vi "Control - Generic - Port Injection Basic Host.vi"() -> ()   [LabVIEW 2015, in "ECS-Host.lvlib"]
uses:
  ECS-Host.lvlib
  <vilib>/addons/Software Calibration Management/XControls/TBL2D.xctl
panel:
  out "InjAdv_Des":sgl[](array[numeric]) caption="[DBTDC]"
  out "InjAdv_TblOut":sgl caption="[DBTDC]"
  in  "CylFuelSplit":sgl[](array[numeric]) caption="[%]"
  in  "InjQty_ManE":bool caption="Enable Inj"
  in  "InjQty_Man":sgl caption="[mg/cyc]"
  in  "InjAdv_ManE":bool caption="Enable Inj"
  in  "InjAdv_Man":sgl caption="[DBTDC]"
  in  "InjAdv_Tbl":cluster{"X":sgl[], "Y":sgl[], "Z":sgl[][]}(xcontrol) caption="[RPM|bar|DBTDC]"
  out "_FuelPulseWidth Cyl Index":string[](array[string]) caption="[]"
  out "InjQty_Des":sgl[](array[numeric]) caption="[mg/cyc]"
  # "Manual Control\n(all cylinders)"
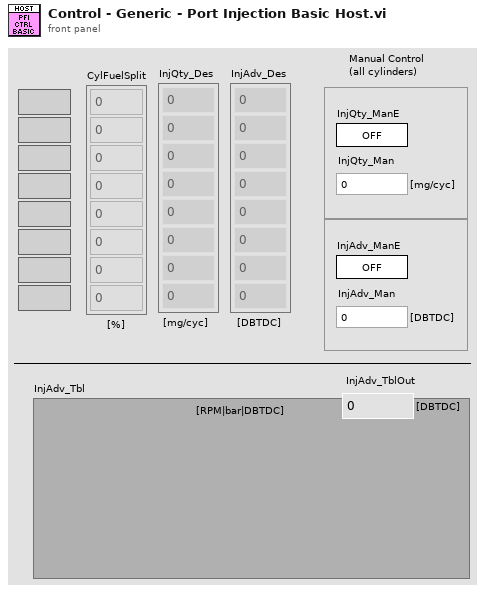
[diagram p1: front panel]
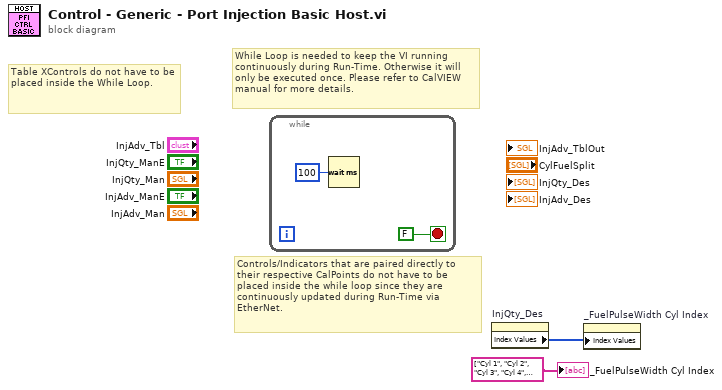
[diagram p0: block diagram]
diagram:
  # "Controls/Indicators that are paired directly to their respective CalPoints do not have to be placed inside the while loop since they are continuously updated during Run-Time via EtherNet."
  # "Table XControls do not have to be placed inside the While Loop."
  # "While Loop is needed to keep the VI running\ncontinuously during Run-Time. Otherwise it will only be executed once. Please refer to CalVIEW manual for more details."
  n1 = while {
    stop <- FALSE stop-if-true
    n2 = Wait (ms)(milliseconds to wait=u32 100) -> ()  [unwired: 1 out]
  }
  n3 = property on="InjQty_Des" class="Arr (strict)"() -> ("Index Values"=w1:u32[])  [unwired: 2 in, 2 out]
  n4 = property on="_FuelPulseWidth Cyl Index" class="Arr (strict)"("Index Values"=w1) -> ()  [unwired: 2 in, 2 out]
  "_FuelPulseWidth Cyl Index" <- string[] ["Cyl 1", "Cyl 2", "Cyl 3", "Cyl 4", "Cyl 5", "Cyl 6", "Cyl 7", "Cyl 8"] ("FuelPulseWidth 3")
